vi "Generate log file path.vi"(8 "error in":errorcluster) -> (0 "error out":errorcluster, 3 "Log File Cluster":T1)   [LabVIEW 2016]
uses:
  Tests/Log File Cluster.ctl
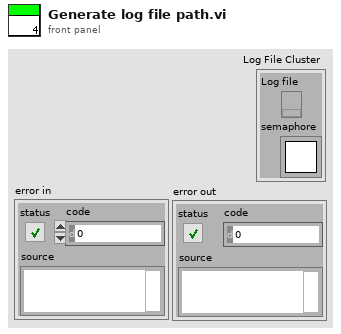
[diagram p1: front panel]
types:
  T1 = typedef "Log File Cluster.ctl" = cluster{"Log file":refnum<k34>, "semaphore":T2}
  T2 = typedef "Semaphore RefNum" = refnum<k1>
  T3 = enum16{"open", "open or create", "create or replace", "create", "open (read-only)"}
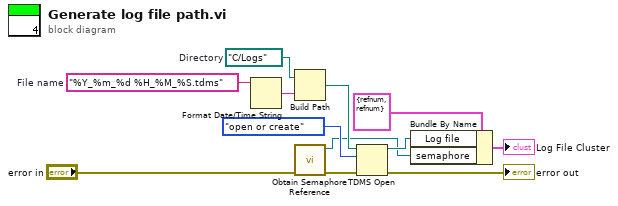
[diagram p0: block diagram]
diagram:
  w7 = path "C:/Logs"  # Directory
  w12 = "%Y_%m_%d %H_%M_%S.tdms"  # File name
  n1 = Format Date/Time String(time format string (%c)=w12) -> (date/time string=w11:string)  [unwired: 2 in]
  n2 = Build Path(base path=w7, name or relative path=w11) -> (appended path=w10:path)
  n3 = call <vilib>:"Obtain Semaphore Reference.vi"("error in (no error)"="error in") -> ("error out"=w5:errorcluster, "semaphore"=w1:T2)  [unwired: 4 in, 1 out]
  n4 = TDMS Open(8:w5, 10:T3."open or create" ("operation (0:open)"), 11:w10) -> (0:→"error out":errorcluster, 3:w2:refnum<k34>)  [unwired: 4 in]
  n5 = Bundle By Name(cluster=T1 {"Log file"=refnum, "semaphore"=refnum} ("Log File Cluster"), "Log file"=w2, "semaphore"=w1) -> (→"Log File Cluster":T1)
